vi "Rysowanie strzałki pod zadanym kątem.vi"(9 "Parametry strzałki":T1={"Położenie grotu"={"Pixel x"=0, "Pixel y"=0}, "Kolor"=0, "Długość [px]"=26, "Kąt/azymut"=2.0, "Interpretacją kąta ustawienia strzałki"=enum."Kąt trygonometryczny", "Grubość"=2, "Długość grotu"=10}, 10 "Zoom mapy":dbl=1.0, 11 "Mapa terenu":picture) -> (3 "Mapa ze strzałką":picture)   [LabVIEW 2012]
doc: "Dorysowanie strzałki do mapy o zadanych parametrach(kolor, długość strzalki i grotu, położenie końca grotu, kąt trygonometryczny lub azymut jako kąt pod którym ustawiona jest strzałka)."
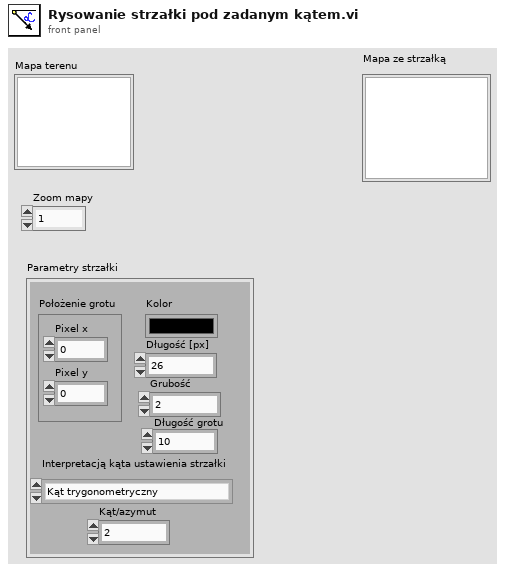
[diagram p1: front panel]
types:
  T1 = cluster{"Położenie grotu":cluster{"Pixel x":i16, "Pixel y":i16}, "Kolor":u32, "Długość [px]":u32, "Kąt/azymut":dbl, "Interpretacją kąta ustawienia strzałki":enum16{"Kąt trygonometryczny", "Azymut"}, "Grubość":u32, "Długość grotu":u32}
  T2 = cluster{"Położenie końca":cluster{"Pixel x":i16, "Pixel y":i16}, "Kolor":u32, "Długość [px]":u32, "Kąt/azymut":dbl, "Interpretacją kąta ustawienia strzałki":enum16{"Kąt trygonometryczny", "Azymut"}, "Grubość":u32}
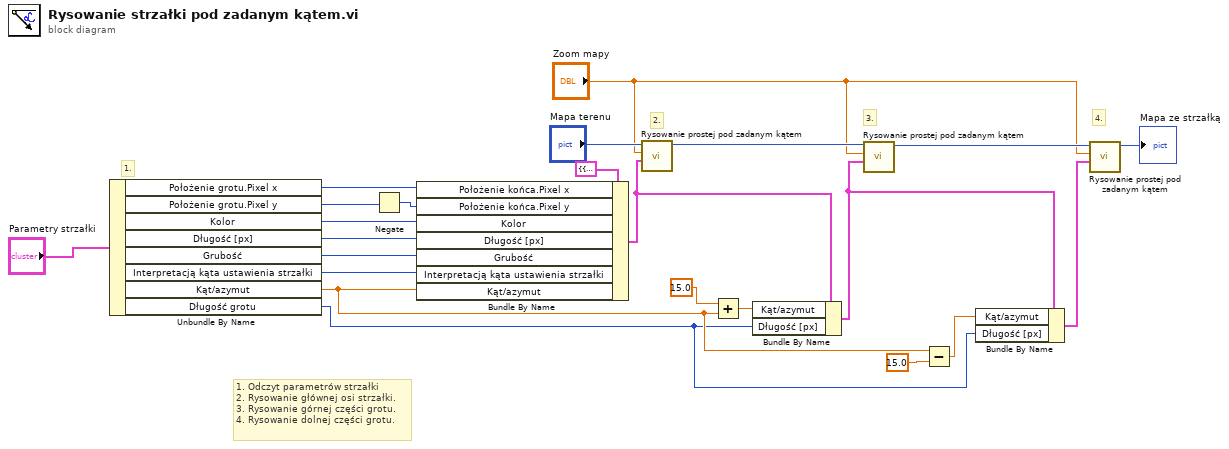
[diagram p0: block diagram]
diagram:
  # "1. Odczyt parametrów strzałki\n2. Rysowanie głównej osi strzałki.\n3. Rysowanie górnej części grotu.\n4. Rysowanie dolnej części grotu."
  # "4."
  # "3."
  # "2."
  # "1."
  n1 = Unbundle By Name("Parametry strzałki") -> ("Położenie grotu.Pixel x"=w3:i16, "Położenie grotu.Pixel y"=w2:i16, "Kolor"=w15:u32, "Długość [px]"=w14:u32, "Grubość"=w13:u32, "Interpretacją kąta ustawienia strzałki"=w12:enum16{"Kąt trygonometryczny", "Azymut"}, "Kąt/azymut"=w6:dbl, "Długość grotu"=w5:u32)
  n2 = Negate(x=w2) -> (-x=w4:i16)
  n3 = Bundle By Name(cluster=T2 {"Położenie końca"={"Pixel x"=55, "Pixel y"=50}, "Kolor"=11811328, "Długość [px]"=26, "Kąt/azymut"=54.0, "Interpretacją kąta ustawienia strzałki"=enum."Azymut", "Grubość"=2} ("Parametry prostej"), "Położenie końca.Pixel x"=w3, "Położenie końca.Pixel y"=w4, "Kolor"=w15, "Długość [px]"=w14, "Grubość"=w13, "Interpretacją kąta ustawienia strzałki"=w12, "Kąt/azymut"=w6) -> (w11:T2)
  n4 = call "Rysowanie prostej pod zadanym kątem.vi"("Parametry prostej"=w11, "Zoom mapy"="Zoom mapy", "Mapa terenu"="Mapa terenu") -> ("Mapa z narysowaną prostą"=w21:picture)  [unwired: 8 in]
  n5 = Add(x=15.0 ("y"), y=w6) -> (x+y=w10:dbl)
  n6 = Bundle By Name(cluster=w11, "Kąt/azymut"=w10, "Długość [px]"=w5) -> (w7:T2)
  n7 = call "Rysowanie prostej pod zadanym kątem.vi"("Parametry prostej"=w7, "Zoom mapy"="Zoom mapy", "Mapa terenu"=w21) -> ("Mapa z narysowaną prostą"=w22:picture)  [unwired: 8 in]
  n8 = Subtract(x=w6, y=15.0) -> (x-y=w19:dbl)
  n9 = Bundle By Name(cluster=w7, "Kąt/azymut"=w19, "Długość [px]"=w5) -> (w8:T2)
  n10 = call "Rysowanie prostej pod zadanym kątem.vi"("Parametry prostej"=w8, "Zoom mapy"="Zoom mapy", "Mapa terenu"=w22) -> ("Mapa z narysowaną prostą"=→"Mapa ze strzałką":picture)  [unwired: 8 in]
